vi "fsk.vi"() -> ()   [LabVIEW 2014]
uses:
  <vilib>/Analysis/NI_AALPro.lvlib
panel:
  out "demod":dynamicdata(graph)
  out "modul":dynamicdata(graph)
  out "dig.data":dbl[](graph)
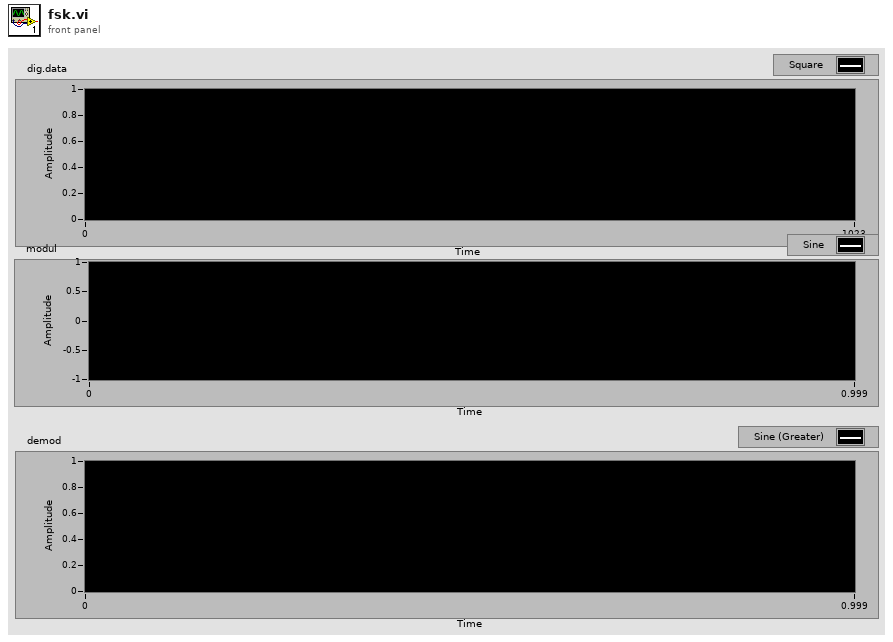
[diagram p1: front panel]
types:
  T1 = enum16{"sine", "cosine", "triangle", "square", "sawtooth", "increasing ramp", "decreasing ramp"}
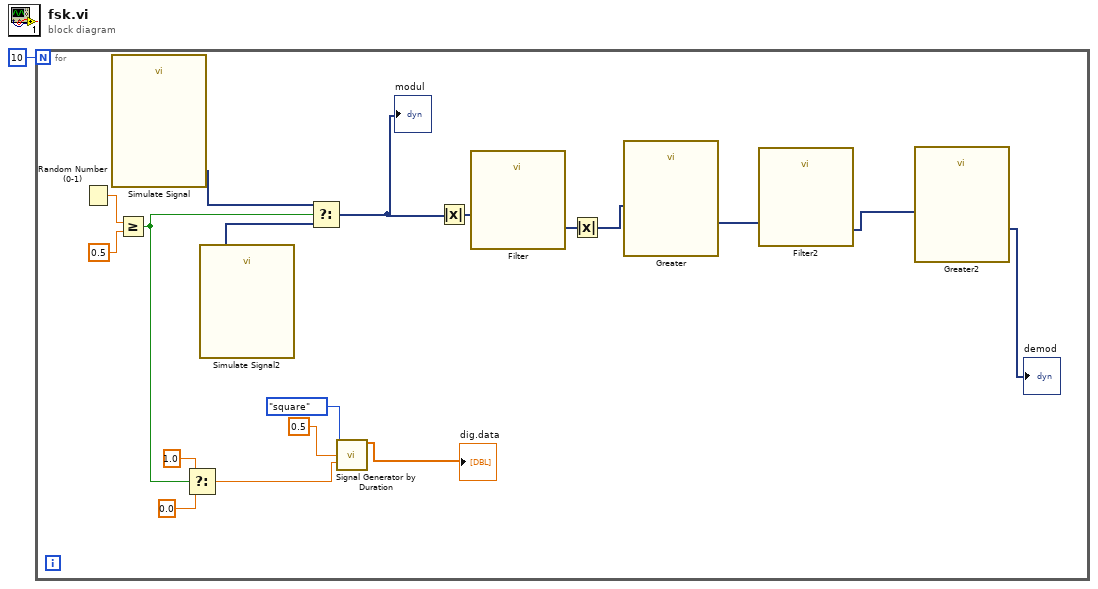
[diagram p0: block diagram]
diagram:
  n1 = for {
    N: 10 -> [_]
    n2 = Random Number (0-1)() -> (number: 0 to 1=w19:dbl)
    n3 = call "Simulate Signal"() -> ("Sine"=w15:dynamicdata)  [unwired: 14 in, 1 out]
    n4 = Greater Or Equal?(x=w19, y=0.5) -> (x >= y?=w13:bool)
    n5 = Select(t=1.0, s=w13, f=0.0) -> (s? t:f=w10:dbl)
    n6 = call "Simulate Signal2"() -> ("Sine"=w14:dynamicdata)  [unwired: 14 in, 1 out]
    n7 = Select(t=w15, s=w13, f=w14) -> (s? t:f=w8:dynamicdata)
    "modul" <- w8
    n8 = call <vilib>:"Signal Generator by Duration.vi"("signal type"=T1."square", "frequency"=0.5, "amplitude"=w10) -> ("signal"=→"dig.data":dbl[])  [unwired: 9 in, 3 out]
    n9 = Absolute Value(x=w8) -> (abs(x)=w7:dynamicdata)
    n10 = call "Filter"("Signal"=w7) -> ("Filtered Signal"=w6:dynamicdata)  [unwired: 9 in, 1 out]
    n11 = Absolute Value(x=w6) -> (abs(x)=w5:dynamicdata)
    n12 = call "Greater"("Operand 1"=w5) -> ("Result"=w4:dynamicdata)  [unwired: 9 in, 1 out]
    n13 = call "Filter2"("Signal"=w4) -> ("Filtered Signal"=w3:dynamicdata)  [unwired: 9 in, 1 out]
    n14 = call "Greater2"("Operand 1"=w3) -> ("Result"=→"demod":dynamicdata)  [unwired: 9 in, 1 out]
  }
